vi "chirp.vi"(7 "LVWSR":refnum<class "Web Request.lvclass">, 10 "fcenter":i16, 11 "df":i16) -> ()   [LabVIEW 2016]
uses:
  <vilib>/wsapi/Web Request.lvclass
  Controller/Messages/Forward Command/Forward Command MSG.lvclass
  C:/Program Files (x86)/National Instruments/LabVIEW 2016/vi.lib/ActorFramework/Message/Message.lvclass
  PAS/Commands/Update Chirp Cmd/Update Chirp CMD.lvclass
  C:/Program Files (x86)/National Instruments/LabVIEW 2016/vi.lib/MSR Consulting, LLC/General Reuse/Command/Command.lvclass
  PAS/Commands/Update Chirp Cmd/Update Chirp CMD.lvclass/Update Chirp CMD.ctl
  Controller/Messages/Forward Command/Forward Command MSG.lvclass/Forward Command MSG.ctl
  <vilib>/ActorFramework/Message Enqueuer/Message Enqueuer.lvclass/Message Enqueuer.ctl
  PAS/Commands/Update Chirp Cmd/Write df.vi
  PAS/Commands/Update Chirp Cmd/Write fcenter.vi
  Controller/Messages/Forward Command/Write id.vi
  Controller/Messages/Forward Command/Write CMD.vi
  <vilib>/ActorFramework/Message Priority Queue/Priority Enqueue.vi
  Controller/gController.lvclass
  <vilib>/ActorFramework/Message Enqueuer/Message Enqueuer.lvclass
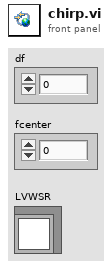
[diagram p1: front panel]
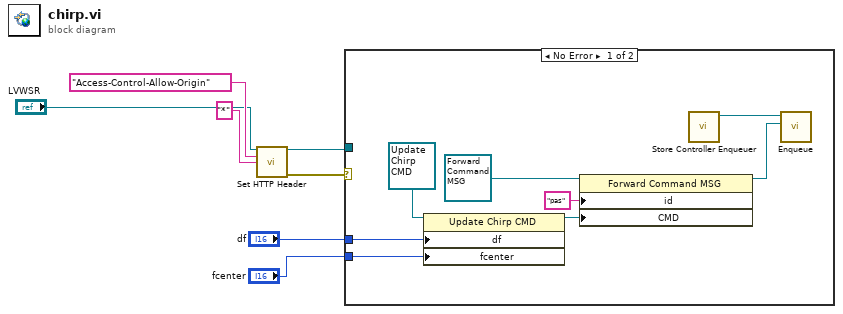
[diagram p0: block diagram]
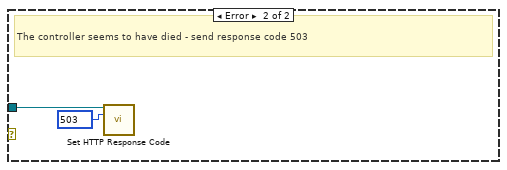
[diagram p2: hidden frame]
diagram:
  n1 = call <vilib>:"Set HTTP Header.vi"("LabVIEW Web Service Request"="LVWSR", "header"="Access-Control-Allow-Origin", "header value"="*") -> ("LabVIEW Web Service Request out"=w2:refnum<class "Web Request.lvclass">, "error out"=w1:errorcluster)  [unwired: 11 in]
  n2 = case shown="No Error" w1 {
    tunnel: w2 -> [_ w16]
    tunnel: "df" -> [w9 _]
    tunnel: "fcenter" -> [w8 _]
    frame No Error {
      n3 = property class="Update Chirp CMD"(reference=refnum<class "Update Chirp CMD.lvclass"> refnum ("gPAS Library.lvlib:Update Chirp CMD"), "df"=w9, "fcenter"=w8) -> (reference out=w10:refnum<class "Update Chirp CMD.lvclass">)  [unwired: 1 in, 1 out]
      n4 = property class="Forward Command MSG"(reference=refnum<class "Forward Command MSG.lvclass"> refnum ("Controller.lvlib:Forward Command MSG.lvclass"), "id"="pas", "CMD"=w10) -> (reference out=w13:refnum<class "Forward Command MSG.lvclass">)  [unwired: 1 in, 1 out]
      n5 = call "Store Controller Enqueuer.vi"() -> ("Controller Enqueuer Out"=w15:refnum<class "Message Enqueuer.lvclass">)  [unwired: 11 in]
      n6 = call <vilib>:"Enqueue.vi"("Message"=w13, "Message Enqueuer in"=w15) -> ()  [unwired: 8 in, 2 out]
    }
    frame Error {
      w17 = 503 items=["100"=100, "101"=101, "200"=200, "201"=201, "202"=202, "203"=203, "204"=204, "205"=205, "206"=206, "300"=300, "301"=301, "302"=302, "303"=303, "304"=304, "305"=305, "306"=306, "307"=307, "400"=400, "401"=401, "402"=402, "403"=403, "404"=404, "405"=405, "406"=406, "407"=407, "408"=408, "409"=409, "410"=410, "411"=411, "412"=412, "413"=413, "414"=414, "415"=415, "416"=416, "417"=417, "500"=500, "501"=501, "502"=502, "503"=503, "504"=504, "505"=505] ("response code (200)")
      # "The controller seems to have died - send response code 503"
      n7 = call <vilib>:"Set HTTP Response Code.vi"("LabVIEW Web Service Request"=w16, "response code (200)"=w17) -> ()  [unwired: 12 in, 2 out]
    }
  }
